vi "Configuration 1.1 Finalize.vi"(8 "error in (no error)":errorcluster, 10 "dsf version (1.1)":T2={"major"=1, "minor"=1, "fix"=0, "build"=""}, 11 "framework configuration 1.1":T1={"plugins"=[{"name"="Plugin", "components"=[], "cycle timing"={"priority"=10000, "decimation"=1, "offset"=0}, "threads"=[], "transfer groups"=[{"name"="Group", "direction"=0, "cycle timing"={"priority"=100, "decimation"=1, "offset"=0}, "thread index"=-1, "settings"=[], "transfers"=[{"name"="Transfer", "byte order"=0, "settings"=[], "channels"=[{"string offset"=0, "string data type"=2, "engine data type"=2, "name"="Channel", "settings"=[], "units"="V"}]}], "timeout behavior"=0}], "settings"=[]}]}) -> (0 "error out":errorcluster, 2 "final dsf version":T2, 3 "dsf configuration json":string)   [LabVIEW 2021, in "DSF Core.lvlib" / "Configuration Session.lvclass"]
uses:
  Configuration Session.lvclass
  Typedefs/DSF Version Info.ctl
  DSF Core.lvlib
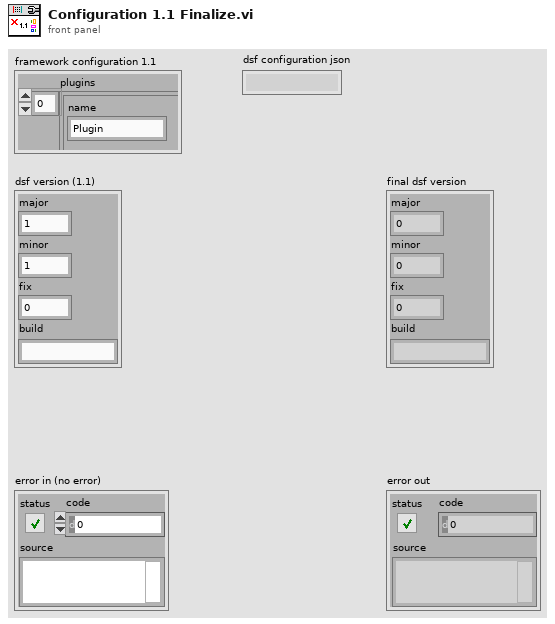
[diagram p1: front panel]
types:
  T1 = cluster{"plugins":cluster{"name":string, "components":string[], "cycle timing":cluster{"priority":u64, "decimation":u64, "offset":u64}, "threads":cluster{"buffer converter settings":cluster{"key":string, "value":string}[], "transceiver settings":cluster{"key":string, "value":string}[], "custom settings":cluster{"key":string, "value":string}[], "processor":i32, "priority offset":i16}[], "transfer groups":cluster{"name":string, "direction":u8, "cycle timing":cluster{"priority":u64, "decimation":u64, "offset":u64}, "thread index":i32, "settings":cluster{"key":string, "value":string}[], "transfers":cluster{"name":string, "byte order":u8, "settings":cluster{"key":string, "value":string}[], "channels":cluster{"string offset":u64, "string data type":u8, "engine data type":u8, "name":string, "settings":cluster{"key":string, "value":string}[], "units":string}[]}[], "timeout behavior":u8}[], "settings":cluster{"key":string, "value":string}[]}[]}
  T2 = typedef "DSF Core.lvlib/DSF Version Info.ctl" = cluster{"major":u32, "minor":u32, "fix":u32, "build":string}
  T3 = cluster{"plugins":cluster{"id":string, "values":cluster{"components":string[], "timing":cluster{"priority":u64, "decimation":u64, "offset":u64}, "group ids":string[], "settings id":string, "threads":cluster{"buffer converter settings":cluster{"key":string, "value":string}[], "transceiver settings":cluster{"key":string, "value":string}[], "custom settings":cluster{"key":string, "value":string}[], "processor":i32, "priority offset":i16}[]}}[], "groups":cluster{"id":string, "values":cluster{"direction":i32, "timing":cluster{"priority":u64, "decimation":u64, "offset":u64}, "transfer ids":string[], "settings id":string, "thread":i32, "timeout behavior":u8}}[], "transfers":cluster{"id":string, "values":cluster{"byte order":i32, "channel ids":string[], "settings id":string}}[], "channels":cluster{"id":string, "values":cluster{"string buffer offset":u64, "string data type":i32, "engine data type":i32, "settings id":string, "units":string}}[], "settings":cluster{"id":string, "values":cluster{"key":string, "value":string}[]}[]}
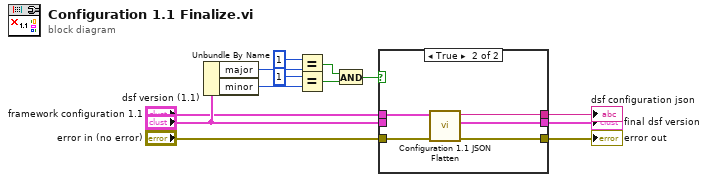
[diagram p0: block diagram]
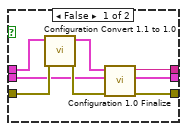
[diagram p2: hidden frame]
diagram:
  n1 = Unbundle By Name("dsf version (1.1)") -> ("major"=w12:u32, "minor"=w13:u32)
  n2 = Equal?(x=u32 1, y=w12) -> (x = y?=w8:bool)
  n3 = Equal?(x=u32 1, y=w13) -> (x = y?=w9:bool)
  n4 = And(x=w8, y=w9) -> (x .and. y?=w7:bool)
  n5 = case shown="True" w7 {
    tunnel: "error in (no error)" -> [w18 w26]
    tunnel: "framework configuration 1.1" -> [w14 w25]
    tunnel: [w21 w24] -> w4
    tunnel: "dsf version (1.1)" -> [w15 _]
    tunnel: [w20 w23] -> w5
    tunnel: [w19 w22] -> w2
    frame False {
      n6 = call "Configuration Convert 1.1 to 1.0.vi"("error in (no error)"=w18, "framework configuration 1.1"=w14) -> ("error out"=w16:errorcluster, "framework configuration 1.0"=w17:T3)  [unwired: 8 in]
      n7 = call "Configuration 1.0 Finalize.vi"("error in (no error)"=w16, "dsf version (1.0)"=w15, "framework configuration 1.0"=w17) -> ("error out"=w21:errorcluster, "final dsf version"=w19:T2, "dsf configuration json"=w20:string)  [unwired: 6 in]
    }
    frame True {
      n8 = call "Configuration 1.1 JSON Flatten.vi"("error in (no error)"=w26, "framework configuration 1.1"=w25) -> ("error out"=w24:errorcluster, "dsf version"=w22:T2, "dsf configuration json"=w23:string)  [unwired: 7 in]
    }
  }
  "dsf configuration json" <- w5
  "error out" <- w4
  "final dsf version" <- w2
